vi "Ophir InitCom.vi"(1 "Baud Rate (3:9600)":i16(ring)=4 items=["300", "1200", "4800", "9600", "19200", "38400"], 2 "error in (no error)":errorcluster, 4 "Port Number (default 2)":i16=1 min=0 max=20, 5 "GPIB Address (default 10)":string="10", 7 "USB Channel number (default 0)":dbl, 8 "Communication (default USB 0)":i16(ring) items=["USB", "RS232", "GPIB"]) -> (0 "error out":errorcluster, 3 "dup Visa Session":refnum<visa-resource-name>, 9 "Visa Session":refnum<visa-resource-name>)   [LabVIEW 2017]
doc: "InitCom.vi initializes the communication with Device\nreturns the VISA Session. \n\nLast Updated 16 May 2010\n\nYou must run this VI before using any of the instrument driver VIs for this instrument.\n\nYou must choose Communication Protocol : USB , RS232 or GPIB\nwhen USB is default.\n\nFor RS232 Protocol you must fill the Port Number and the Baud Rate.\n\nInputs:\nUSB,RS232,GPIB:Communication\nSelect Protocol USB(0) , RS232(1) or GPIB(2)\nDefault 0:USB\n\nUSB Channel number\nDefault: 0\n\nGPIB Address:\nString defaut:10 for LS Device\n\nPort Number\nThe Port Number control specifies the serial port .\nPort Number 1 corresponds to serial port 1, Port Number 2 = serial port 2, etc.\ndefault: 2\n\nBaud Rate :\n0:300 bps\n1:1200 bps\n2:4800 bps\n3:9600 bps\n4:19200 bps\n5:38400 bps\ndefault: 3:9600 bps\n\nOutputs:\ndup Visa Session\nErrorOut\n\nNote:\nThe Device fixed communication parameters are:\nData bits:8\nStop bits:1\nParity:None"
panel:
  # "PC:  1 = COM1, 2= COM2,.."
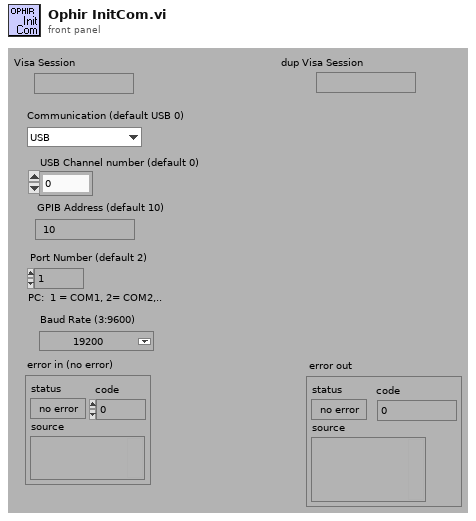
[diagram p1: front panel]
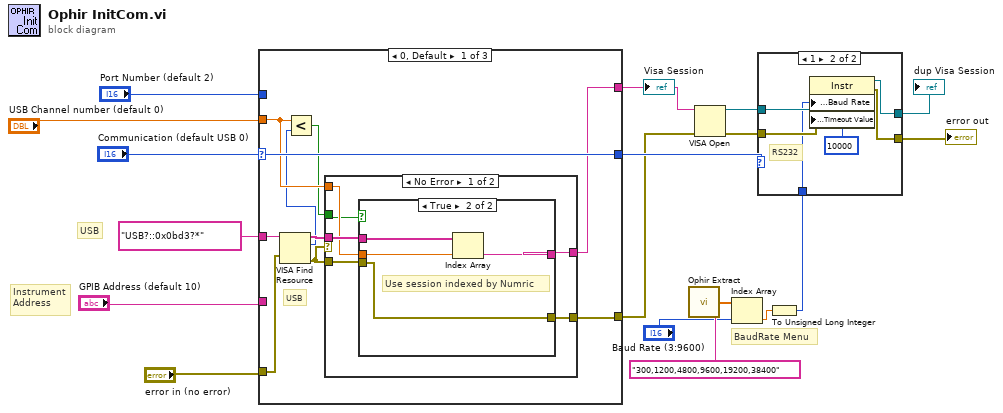
[diagram p0: block diagram]
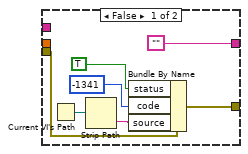
[diagram p2: hidden frame]
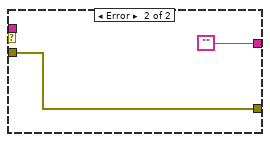
[diagram p3: hidden frame]
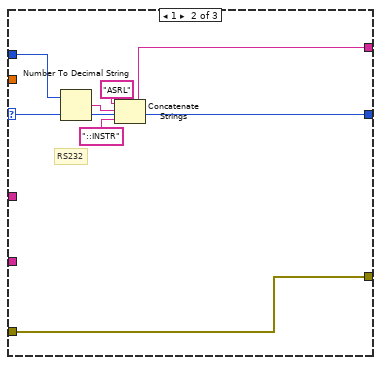
[diagram p4: hidden frame]
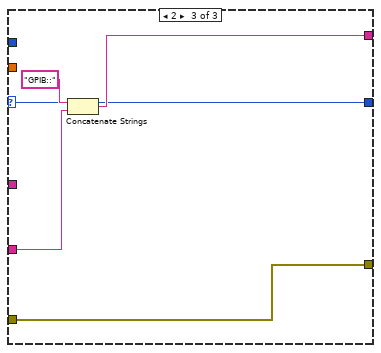
[diagram p5: hidden frame]
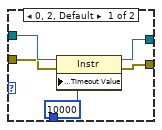
[diagram p6: hidden frame]
diagram:
  # "USB"
  # "Instrument\nAddress"
  # "BaudRate Menu"
  n1 = case shown="0, Default" "Communication (default USB 0)" {
    selector: "Communication (default USB 0)" -> [w26 w50 w57]
    tunnel: [w21 w51 w58] -> w8
    tunnel: [w26 w50 w57] -> w15
    tunnel: "Port Number (default 2)" -> [_ w48 _]
    tunnel: "GPIB Address (default 10)" -> [_ _ w56]
    tunnel: "USB?::0x0bd3?*" ("USB0::0x0BD3") -> [w28 _ _]
    tunnel: "error in (no error)" -> [w27 w49 w55]
    tunnel: [w25 w49 w55] -> w4
    tunnel: "USB Channel number (default 0)" -> [w22 _ _]
    frame 0, Default {
      # "USB"
      n2 = VISA Find Resource(8:w27, 11:w28) -> (0:w23:errorcluster, 2:w19:u32, 3:w24:string[])  [unwired: 1 out]
      n3 = Less?(x=w22, y=w19) -> (x < y?=w20:bool)
      n4 = case shown="No Error" w23 {
        tunnel: [w29 w47] -> w25
        tunnel: w24 -> [w34 _]
        tunnel: w23 -> [w33 w47]
        tunnel: w22 -> [w32 _]
        tunnel: [w31 ""] -> w21
        tunnel: w20 -> [w30 _]
        frame No Error {
          n5 = case shown="True" w30 {
            tunnel: w34 -> [_ w45]
            tunnel: ["" w44] -> w31
            tunnel: w32 -> [_ w43]
            tunnel: w33 -> [w39 w42]
            tunnel: [w35 w42] -> w29
            frame False {
              n6 = Current VI's Path() -> (path=w40:path)
              n7 = Strip Path(path=w40) -> (name=w38:string)  [unwired: 1 out]
              n8 = Bundle By Name(cluster=w39, "status"=TRUE, "code"=-1341, "source"=w38) -> (w35:errorcluster)
            }
            frame True {
              # "Use session indexed by Numric"
              n9 = Index Array(array=w45, index=w43) -> (element=w44:string)
            }
          }
        }
        frame Error {
        }
      }
    }
    frame 1 {
      # "RS232"
      n10 = Number To Decimal String(number=w48) -> (decimal integer string=w52:string)  [unwired: 1 out]
      n11 = Concatenate Strings("ASRL", w52, "::INSTR") -> (w51:string)
    }
    frame 2 {
      n12 = Concatenate Strings("GPIB::", w56) -> (w58:string)
    }
  }
  "Visa Session" <- w8
  n13 = call "Ophir Extract.vi"("String"="300,1200,4800,9600,19200,38400") -> ("Single Precision Array"=w12:sgl[])
  n14 = VISA Open(error in (no error)=w4, VISA resource name=w8) -> (VISA resource name=w18:refnum<visa-resource-name>, error out=w14:errorcluster)  [unwired: 3 out]
  n15 = Index Array(array=w12, index="Baud Rate (3:9600)") -> (element=w10:sgl)
  n16 = To Unsigned Long Integer(number=w10) -> (unsigned 32bit integer=w9:u32)
  n17 = case shown="1" w15 {
    tunnel: w18 -> [w64 w70]
    tunnel: [w63 w69] -> w17
    tunnel: [w61 w67] -> w16
    tunnel: w14 -> [w62 w68]
    tunnel: w9 -> [_ w66]
    frame 0, 2, Default {
      n18 = property class="Instr"(reference=w64, error in=w62, "General Settings:Timeout Value"=u32 10000) -> (reference out=w63:refnum<visa-resource-name>, error out=w61:errorcluster)
    }
    frame 1 {
      # "RS232"
      n19 = property class="Instr"(reference=w70, error in=w68, "Serial Settings:Baud Rate"=w66, "General Settings:Timeout Value"=u32 10000) -> (reference out=w69:refnum<visa-resource-name>, error out=w67:errorcluster)
    }
  }
  "error out" <- w16
  "dup Visa Session" <- w17
